vi "DMM Init.vi"(8 "error in (no error)":errorcluster, 10 "Instrument Descriptor":refnum<k15>, 11 "DMM in":refnum<class "DMM.lvclass">) -> (0 "error out":errorcluster, 2 "Instrument out":refnum<k15> caption="instrument handle out", 3 "DMM out":refnum<class "DMM.lvclass">)   [LabVIEW 2023, in "HardwareAbstractionLayer_LVOOP.lvlib" / "DMM.lvclass"]
uses:
  DMM.lvclass
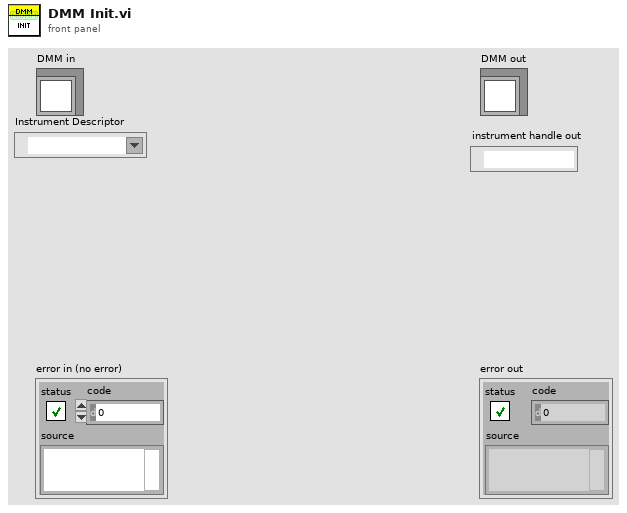
[diagram p1: front panel]
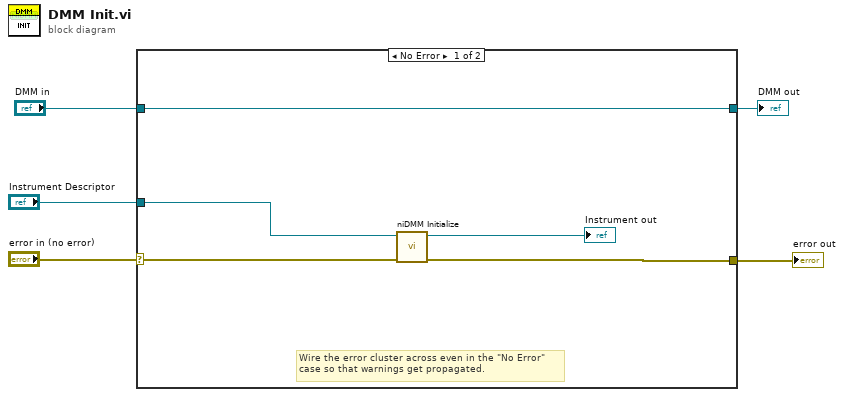
[diagram p0: block diagram]
diagram:
  n1 = case shown="No Error" "error in (no error)" {
    selector: "error in (no error)" -> [w9 w12]
    tunnel: [w8 w12] -> w4
    tunnel: [w10 w11] -> w2
    tunnel: "DMM in" -> [w10 w11]
    tunnel: "Instrument Descriptor" -> [w7 _]
    frame No Error {
      # "Wire the error cluster across even in the \"No Error\"\ncase so that warnings get propagated."
      n2 = call <instrlib>:"niDMM Initialize.vi"("error in (no error)"=w9, "Instrument Descriptor"=w7) -> ("error out"=w8:errorcluster, "instrument handle out"=→"Instrument out":refnum<k15>)  [unwired: 8 in]
    }
    frame Error {
    }
  }
  "error out" <- w4
  "DMM out" <- w2
